vi "Initialize Core.vi"(8 "error in (no error)":errorcluster, 10 "Parameters":refnum<class "Abstract Init Parameters.lvclass">, 11 "Reflected Name Consumer in":refnum<class "Test Consumer.lvclass">) -> (0 "error out":errorcluster, 3 "Reflected Name Consumer out":refnum<class "Test Consumer.lvclass">)   [LabVIEW 2027, in "Test Consumer.lvclass"]
uses:
  Test Consumer.lvclass
  Parameters/Abstract Init Parameters/Abstract Init Parameters.lvclass
  Test Consumer.lvclass/Test Consumer.ctl
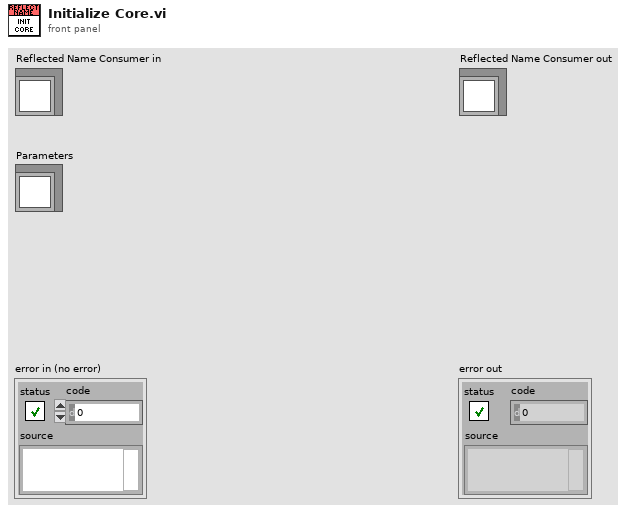
[diagram p1: front panel]
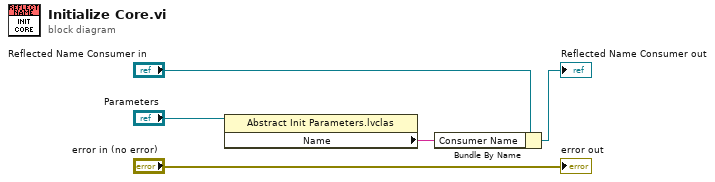
[diagram p0: block diagram]
diagram:
  n1 = property class="Abstract Init Parameters.lvclas"(reference="Parameters") -> ("Name"=w2:string)  [unwired: 1 in, 2 out]
  n2 = Bundle By Name(cluster="Reflected Name Consumer in", "Consumer Name"=w2) -> (→"Reflected Name Consumer out":refnum<class "Test Consumer.lvclass">)
  "error out" <- "error in (no error)"
